vi "Get Absolute Cut Length Positions.vi"(8 "error in (no error)":errorcluster, 10 "Table Stages":T3, 11 "Vibratome":T4) -> (0 "error out":errorcluster, 1 "Pre Cut Dwell [s]":u32, 2 "Slice Position":T3, 3 "Original Position":T3, 4 "Post Cut Dwell [s]":u32, 5 "Slice Axis":enum16{"X Axis", "Y Axis", "Z Axis"}(ring))   [LabVIEW 2017]
uses:
  Hardware/Table Stage/Controls/Translation Stage Cluster.ctl
  Controls/Translation Stage Types.ctl
  Controls/Set Get Controls.ctl
  Hardware/Table Stage/Controls/Motion Translation Module Control.ctl
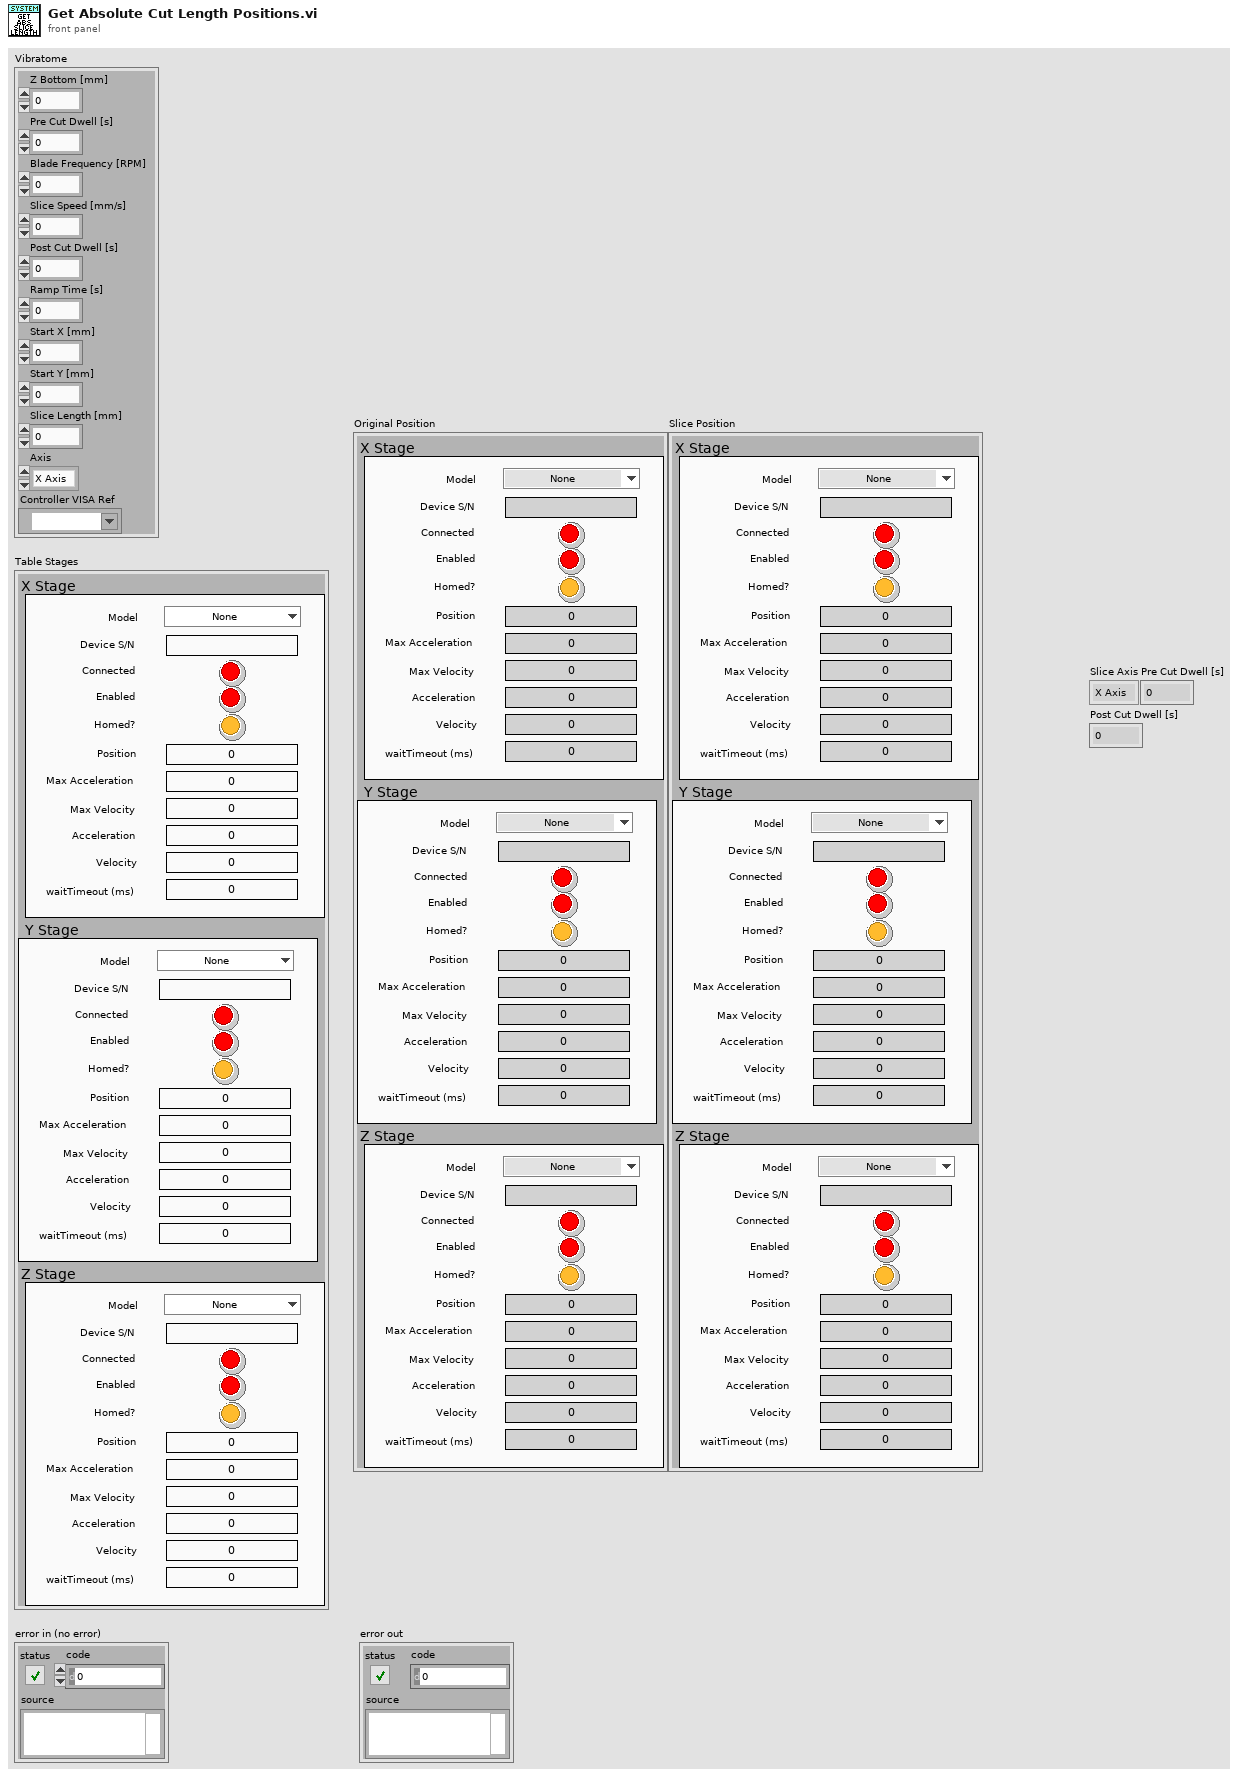
[diagram p1: front panel]
types:
  T1 = typedef "Translation Stage Cluster.ctl" = cluster{"Position":dbl, "Is.Enabled?":bool, "Is.Connected?":bool, "Device SN":string, "AccelerationMaximum":dbl, "VelocityMaximum":dbl, "Acceleration":dbl, "Velocity":dbl, "waitTimeout (ms)":i32, "Model":T2, "Is.Homed?":bool}
  T2 = typedef "Translation Stage Types.ctl" = enum16{"None", "Thorlabs LTS", "Thorlabs MLJ"}
  T3 = cluster{"X Stage":T1, "Y Stage":T1, "Z Stage":T1}
  T4 = cluster{"Z Bottom [mm]":dbl, "Pre Cut Dwell [s]":dbl, "Blade Frequency [RPM]":u16, "Slice Speed [mm/s]":dbl, "Post Cut Dwell [s]":dbl, "Ramp Time [s]":dbl, "Start X [mm]":dbl, "Start Y [mm]":dbl, "Slice Length [mm]":dbl, "Axis":enum16{"X Axis", "Y Axis", "Z Axis"}, "Controller VISA Ref":refnum<visa-resource-name>}
  T5 = typedef "Motion Translation Module Control.ctl" = enum16{"Init", "Home", "Status", "Velocity/Accel", "Position", "Jog", "Stop", "Uninit", "Enable", "Disable"}
  T6 = typedef "Set Get Controls.ctl" = enum16{"Set", "Get"}
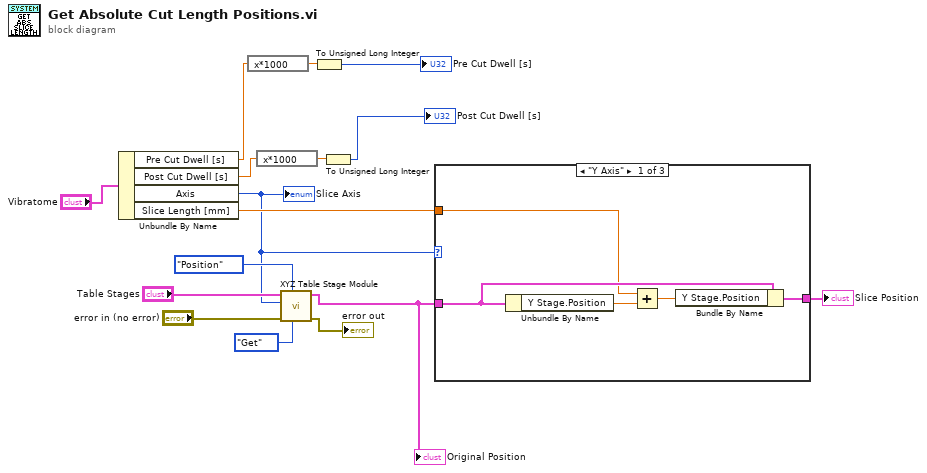
[diagram p0: block diagram]
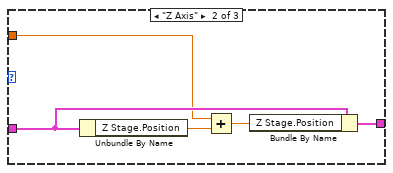
[diagram p2: hidden frame]
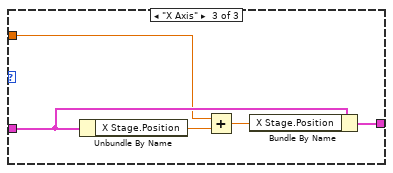
[diagram p3: hidden frame]
diagram:
  n1 = Unbundle By Name("Vibratome") -> ("Pre Cut Dwell [s]"=w5:dbl, "Post Cut Dwell [s]"=w2:dbl, "Axis"=w8:enum16{"X Axis", "Y Axis", "Z Axis"}, "Slice Length [mm]"=w13:dbl)
  "Slice Axis" <- w8
  n2 = expression code="x*1000"(w5) -> (w6:dbl)
  n3 = expression code="x*1000"(w2) -> (w3:dbl)
  n4 = call "XYZ Table Stage Module.vi"("Set/Get"=Set_Get_Controls."Get", "Action"=Motion_Translation_Module_Control."Position", "Error In"="error in (no error)", "Axis"=w8, "Table Stages"="Table Stages") -> ("Error Out"=→"error out":errorcluster, "Table Stages Out"=w16:T3)  [unwired: 5 in]
  "Original Position" <- w16
  n5 = To Unsigned Long Integer(number=w6) -> (unsigned 32bit integer=→"Pre Cut Dwell [s]":u32)
  n6 = To Unsigned Long Integer(number=w3) -> (unsigned 32bit integer=→"Post Cut Dwell [s]":u32)
  n7 = case shown="\"Y Axis\"" w8 {
    tunnel: w16 -> [w21 w26 w31]
    tunnel: w13 -> [w19 w24 w29]
    tunnel: [w17 w22 w27] -> w7
    frame "Y Axis" {
      n8 = Unbundle By Name(w21) -> ("Y Stage.Position"=w18:dbl)
      n9 = Add(x=w19, y=w18) -> (x+y=w20:dbl)
      n10 = Bundle By Name(cluster=w21, "Y Stage.Position"=w20) -> (w17:T3)
    }
    frame "Z Axis" {
      n11 = Unbundle By Name(w26) -> ("Z Stage.Position"=w23:dbl)
      n12 = Add(x=w24, y=w23) -> (x+y=w25:dbl)
      n13 = Bundle By Name(cluster=w26, "Z Stage.Position"=w25) -> (w22:T3)
    }
    frame "X Axis" {
      n14 = Unbundle By Name(w31) -> ("X Stage.Position"=w28:dbl)
      n15 = Add(x=w29, y=w28) -> (x+y=w30:dbl)
      n16 = Bundle By Name(cluster=w31, "X Stage.Position"=w30) -> (w27:T3)
    }
  }
  "Slice Position" <- w7
